vi "Index Objects.vi"(0 "Object List in":i32[][](array[numeric]), 5 "error in (no error)":errorcluster, 7 "index":i32) -> (14 "Object Start/Stop/Sum":i32[](array[numeric]), 19 "error out":errorcluster)   [LabVIEW 2016]
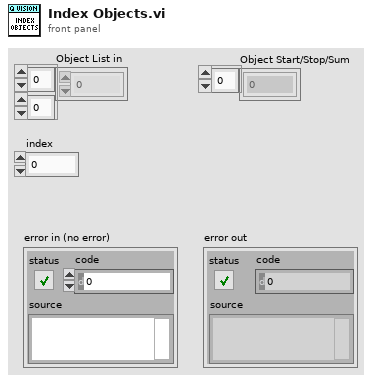
[diagram p1: front panel]
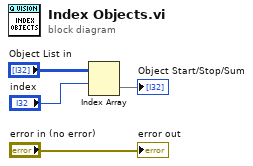
[diagram p0: block diagram]
diagram:
  n1 = Index Array(array="Object List in", index (row)="index") -> (element=→"Object Start/Stop/Sum":i32[])  [unwired: 1 in]
  "error out" <- "error in (no error)"
